vi "ADAPTED_SBG_Ellipse_case_select_n_buffer (SubVI) (1).vi"(6 "new data in":string, 7 "buffer data in":string) -> (0 "case_selector":string, 1 "data out":string, 2 "msg_id":string)   [LabVIEW 2017]
doc: "Filters out unwanted/unneccesary data packets, and sends remaining buffer to case structure to be read. Looks for start bytes FF5A (hex) and consecutive identifiers 03 (Acceleration and Internal Temperature), 13 (Odometer velocity), and 24 (Pressure). Additionally, throws out data that is not readable."
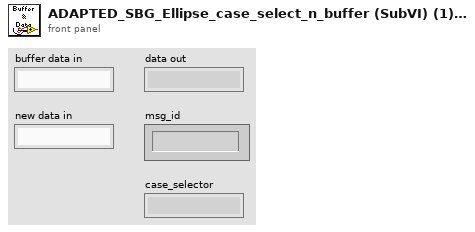
[diagram p1: front panel]
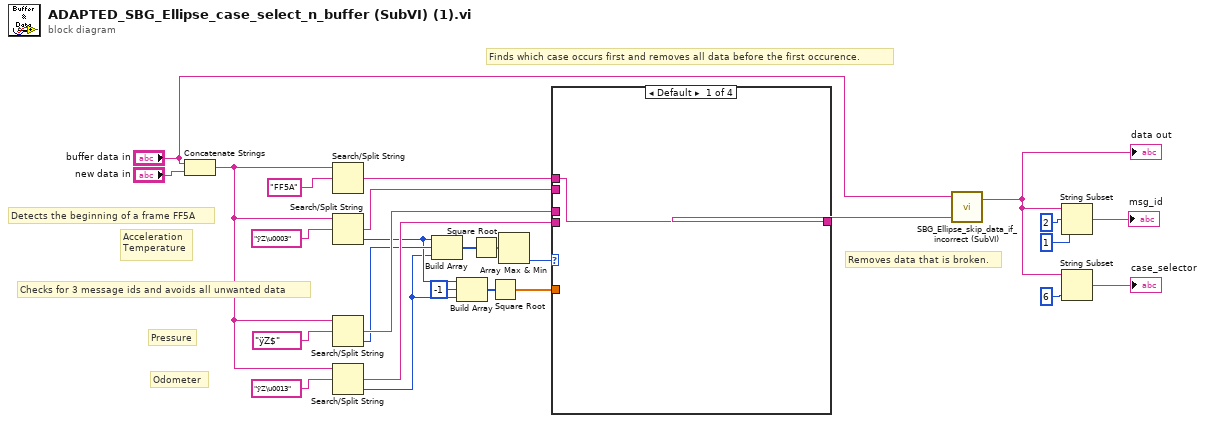
[diagram p0: block diagram]
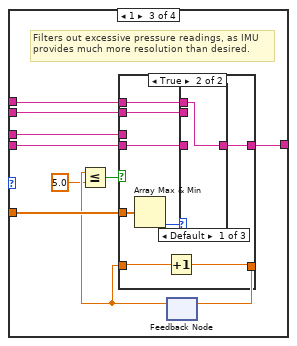
[diagram p3: hidden frame]
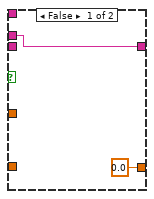
[diagram p4: hidden frame]
diagram:
  # "Removes data that is broken."
  # "Finds which case occurs first and removes all data before the first occurence."
  # "Odometer"
  # "Pressure"
  # "Acceleration\nTemperature"
  # "Checks for 3 message ids and avoids all unwanted data"
  # "Detects the beginning of a frame FF5A"
  n1 = Concatenate Strings("buffer data in", "new data in") -> (w9:string)
  n2 = Search/Split String(string=w9, search string/char (-)="FF5A") -> (match + rest of string=w17:string)  [unwired: 1 in, 2 out]
  n3 = Search/Split String(string=w9, search string/char (-)="ÿZ\u0003") -> (match + rest of string=w20:string, offset of match=w6:i32)  [unwired: 1 in, 1 out]
  n4 = Search/Split String(string=w9, search string/char (-)="ÿZ$") -> (match + rest of string=w19:string, offset of match=w7:i32)  [unwired: 1 in, 1 out]
  n5 = Search/Split String(string=w9, search string/char (-)="ÿZ\u0013") -> (match + rest of string=w8:string, offset of match=w5:i32)  [unwired: 1 in, 1 out]
  n6 = Build Array(w6, w7, w5) -> (w12:i32[])
  n7 = Build Array(w6, -1 ("element"), w5) -> (w3:i32[])
  n8 = Square Root(x=w12) -> (sqrt(x)=w11:dbl[])
  n9 = Square Root(x=w3) -> (sqrt(x)=w2:dbl[])
  n10 = Array Max & Min(array=w11) -> (min index (indices)=w16:i32)  [unwired: 3 out]
  n11 = case shown="Default" w16 {
    tunnel: w20 -> [_ w29 w34 _]
    tunnel: w19 -> [_ _ w38 _]
    tunnel: [w28 w29 w35 w53] -> w15
    tunnel: w17 -> [w28 _ w37 _]
    tunnel: w8 -> [_ _ w36 w53]
    tunnel: w2 -> [_ _ w39 _]
    frame Default {
    }
    frame 0 {
    }
    frame 1 {
      # "Filters out excessive pressure readings, as IMU\nprovides much more resolution than desired."
      n12 = feedback #1() -> (w31:dbl)  [unwired: 1 in]
      n13 = Less Or Equal?(x=w31, y=5.0) -> (x <= y?=w32:bool)
      n14 = case shown="True" w32 {
        tunnel: w39 -> [_ w49]
        tunnel: w38 -> [w41 _]
        tunnel: w37 -> [_ w47]
        tunnel: w36 -> [_ w46]
        tunnel: [w41 w45] -> w35
        tunnel: w34 -> [_ w44]
        tunnel: w31 -> [_ w43]
        tunnel: [0.0 w42] -> w33
        frame False {
        }
        frame True {
          n15 = Array Max & Min(array=w49) -> (min index (indices)=w48:i32)  [unwired: 3 out]
          n16 = Increment(x=w43) -> (x+1=w42:dbl)
          n17 = case shown="Default" w48 {
            tunnel: w47 -> [w50 _ _]
            tunnel: w46 -> [_ _ w52]
            tunnel: [w50 w51 w52] -> w45
            tunnel: w44 -> [_ w51 _]
            frame Default {
            }
            frame 0 {
            }
            frame 2 {
            }
          }
        }
      }
      n18 = feedback-in #1(w33) -> ()
    }
    frame 2 {
    }
  }
  n19 = call "SBG_Ellipse_skip_data_if_incorrect (SubVI).vi"("String"=w15, "result string in"="buffer data in") -> ("result string out"=w13:string)  [unwired: 2 in]
  "data out" <- w13
  n20 = String Subset(string=w13, offset (0)=2, length (rest)=1 ("length (rest)")) -> (substring=→"msg_id":string)
  n21 = String Subset(string=w13, length (rest)=6 ("length (len. of substring)")) -> (substring=→"case_selector":string)  [unwired: 1 in]
